vi "SMC.vi"() -> ()   [LabVIEW 2018]
doc: "PNA-X Example."
uses:
  PNA-X.lvlib
panel:
  out "VISA OUT":refnum<visa-resource-name>
  out "error out":errorcluster
  in  "error in (no error)":errorcluster
  in  "VISA IN":refnum<visa-resource-name>
  out "XY Graph":cluster{"X-Axis":dbl[], "Data":dbl[]}(graph)
  # "1. Select Instrument Source from the \"VISA IN\" drop down.\n2. Run vi"
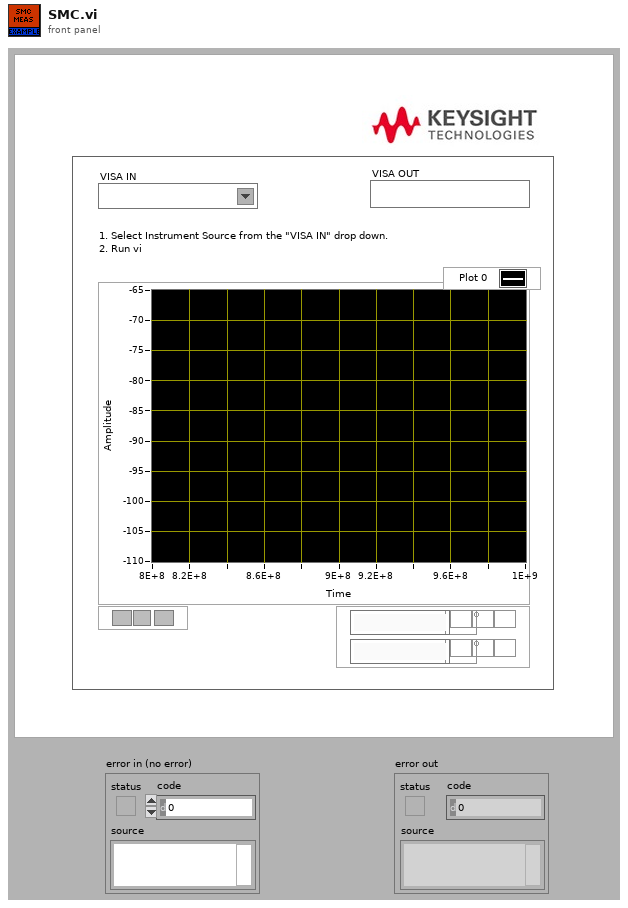
[diagram p1: front panel]
types:
  T1 = cluster{"Mixer Side":string, "Mixer file (*.mxr)":path, "Format":string, "Measurement":string, "OK Button":bool}
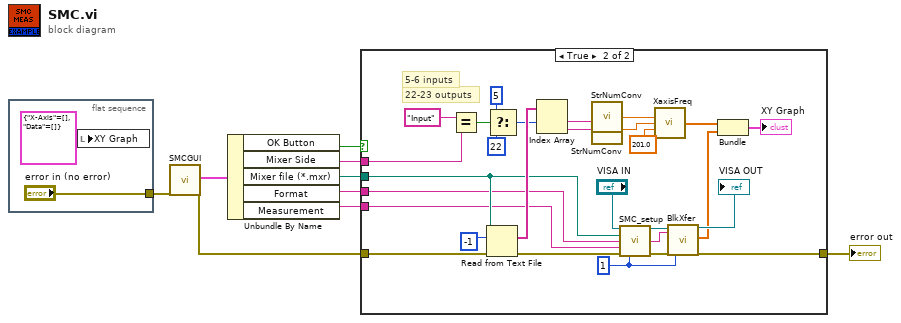
[diagram p0: block diagram]
diagram:
  n1 = flat-sequence {
    tunnel: ["error in (no error)"] -> w8
    frame #0 {
      n2 = local write "XY Graph"(cluster{"X-Axis":dbl[], "Data":dbl[]} {"X-Axis"=[], "Data"=[]} ("XY Graph")) -> ()
    }
  }
  n3 = call "SMCGUI.vi"("error in (no error)"=w8) -> ("output cluster"=w1:T1, "error out"=w6:errorcluster)  [unwired: 17 in]
  n4 = Unbundle By Name(w1) -> ("OK Button"=w7:bool, "Mixer Side"=w5:string, "Mixer file (*.mxr)"=w4:path, "Format"=w3:string, "Measurement"=w2:string)
  n5 = case shown="True" w7 {
    tunnel: [w12 w35] -> w9
    tunnel: w6 -> [w12 w13]
    tunnel: w5 -> [_ w17]
    tunnel: w4 -> [_ w16]
    tunnel: w3 -> [_ w15]
    tunnel: w2 -> [_ w14]
    frame False {
    }
    frame True {
      w34 = 1 ("Channel")
      # "22-23 outputs"
      # "5-6 inputs"
      n6 = Equal?(x="Input", y=w17) -> (x = y?=w32:bool)
      n7 = Read from Text File(file (use dialog)=w16, count=-1, error in=w13) -> (text=w28:string[], error out=w25:errorcluster)  [unwired: 1 in, 2 out]
      n8 = Select(t=5, s=w32, f=22) -> (s? t:f=w27:i32)
      n9 = Index Array(array=w28, index #1=w27) -> (element #1=w21:string, element #2=w19:string)  [unwired: 1 in]
      n10 = call "StrNumConv.vi"("Freq. String"=w21) -> ("Freq."=w20:dbl)  [unwired: 6 in]
      n11 = call "StrNumConv.vi"("Freq. String"=w19) -> ("Freq."=w18:dbl)  [unwired: 6 in]
      n12 = call "SMC_setup.vi"("VISA Resource Name"="VISA IN", "Mixer file (*.mxr)"=w16, "Format"=w15, "Measurement"=w14, "error in (no error)"=w25, "Channel"=w34) -> ("dup VISA session"=w38:refnum<visa-resource-name>, "Filename"=w37:string, "error out"=w39:errorcluster)  [unwired: 7 in]
      n13 = call "XaxisFreq.vi"("Start Frequency"=w20, "Stop Frequency"=w18, "Points"=201.0) -> ("X-Axis"=w24:dbl[])  [unwired: 12 in]
      n14 = call "BlkXfer.vi"("VISA IN"=w38, "FileName"=w37, "error in"=w39, "Channel"=w34) -> ("VISA Out"=→"VISA OUT":refnum<visa-resource-name>, "Data"=w23:dbl[], "error out"=w35:errorcluster)  [unwired: 13 in]
      n15 = Bundle("X-Axis"=w24, "Data"=w23) -> (→"XY Graph":cluster{"X-Axis":dbl[], "Data":dbl[]})  [unwired: 1 in]
    }
  }
  "error out" <- w9
